vi "Test Example Cluster 1.vi"() -> ()   [LabVIEW 2014]
uses:
  <vilib>/Utility/traverseref.llb/TRef TravTarget.ctl
  <vilib>/Utility/traverseref.llb/VI Scripting - Traverse.lvlib
panel:
  out "String":string="struct{}"
  out "ClusterConstant elements datatypes":string[][](array[string])
  out "ClusterConstant TypedefPath":string[](array[string])
  out "All Objects ClassName":string[](array[string])
  in  "vi path":path=path "C:/Users/lubo/Documents/LabView/LabVIEW-Universal-Transcriptor/Test/Examples For Parsing/Example Cluster 1.vi"
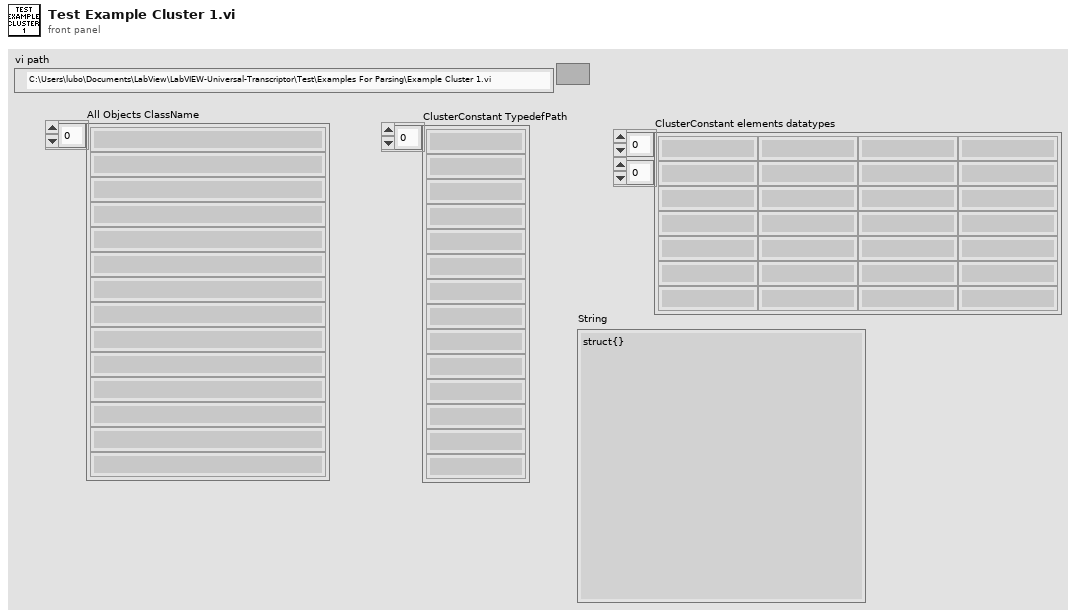
[diagram p1: front panel]
types:
  T1 = typedef "TRef TravTarget.ctl" = enum16{"FP", "BD", "Other"}
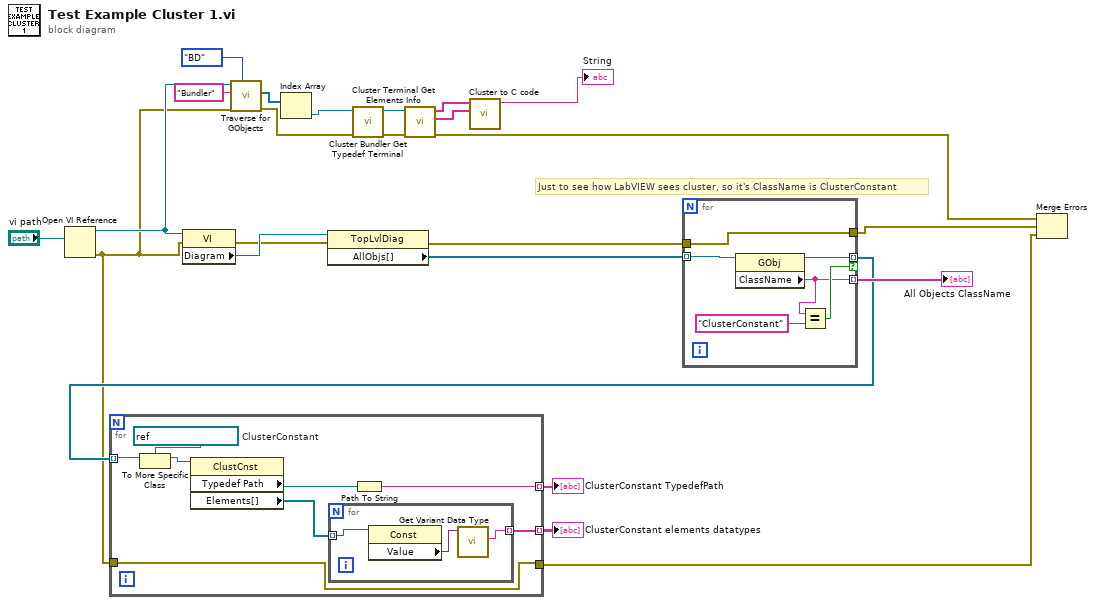
[diagram p0: block diagram]
diagram:
  # "Just to see how LabVIEW sees cluster, so it's ClassName is ClusterConstant"
  n1 = Open VI Reference(vi path="vi path") -> (vi reference=w8:refnum<vi>, error out=w7:errorcluster)  [unwired: 5 in]
  n2 = property class="VI"(reference=w8, error in=w7) -> (error out=w12:errorcluster, "Diagram"=w23:refnum<vi>)  [unwired: 1 out]
  n3 = call <vilib>:"Traverse for GObjects.vi"("Traverse Target"=TRef_TravTarget."BD", "error in (no error)"=w7, "Class Name"="Bundler", "VI Refnum"=w8) -> ("error out"=w6:errorcluster, "References"=w15:refnum<vi>[])  [unwired: 4 in, 2 out]
  n4 = Index Array(array=w15) -> (element=w14:refnum<vi>)  [unwired: 1 in]
  n5 = property class="TopLvlDiag"(reference=w23, error in=w12) -> (error out=w11:errorcluster, "AllObjs[]"=w22:refnum<vi>[])  [unwired: 1 out]
  n6 = call "Cluster Bundler Get Typedef Terminal.vi"("error in (no error)"=w6, "GObject in"=w14) -> ("error out"=w4:errorcluster, "Terminal out"=w13:refnum<vi>)  [unwired: 8 in]
  n7 = call "Cluster Terminal Get Elements Info.vi"("error in (no error)"=w4, "Terminal in"=w13) -> ("error out"=w5:errorcluster, "Cluster elements datatypes"=w2:string[], "Cluster elements names"=w3:string[])  [unwired: 5 in, 2 out]
  n8 = call "Cluster to C code.vi"("Cluster elements datatypes"=w2, "Cluster elements names"=w3) -> ("C code"=→"String":string)  [unwired: 9 in]
  n9 = for {
    tunnel: w22 -> [w30] mode=indexing
    tunnel: [w26] -> w21 mode=indexing
    tunnel: [w28] -> w20 mode=indexing if=w27
    tunnel: [w25] -> w10
    tunnel: w11 -> [w25]
    n10 = property class="GObj"(reference=w30) -> (reference out=w28:refnum<vi>, "ClassName"=w26:string)  [unwired: 1 in, 1 out]
    n11 = Equal?(x=w26, y="ClusterConstant") -> (x = y?=w27:bool)
  }
  "All Objects ClassName" <- w21
  n12 = for {
    tunnel: w20 -> [w38] mode=indexing
    tunnel: [w34] -> w19 mode=indexing
    tunnel: [w32] -> w18 mode=indexing
    tunnel: w7 -> [w31]
    tunnel: [w31] -> w9
    w37 = refnum<vi> refnum  # ClusterConstant
    n13 = To More Specific Class(target class=w37, reference=w38) -> (specific class reference=w36:refnum<vi>)  [unwired: 1 in, 1 out]
    n14 = property class="ClustCnst"(reference=w36) -> ("Typedef Path"=w35:path, "Elements[]"=w33:refnum<vi>[])  [unwired: 1 in, 2 out]
    n15 = for {
      tunnel: w33 -> [w41] mode=indexing
      tunnel: [w39] -> w32 mode=indexing
      n16 = property class="Const"(reference=w41) -> ("Value"=w40:variant)  [unwired: 1 in, 2 out]
      n17 = call "Get Variant Data Type.vi"("Variant in"=w40) -> ("first data type"=w39:string)  [unwired: 9 in, 1 out]
    }
    n18 = Path To String(path=w35) -> (string=w34:string)
  }
  "ClusterConstant TypedefPath" <- w19
  "ClusterConstant elements datatypes" <- w18
  n19 = Merge Errors(w5, w10, w9) -> ()  [unwired: 1 out]
